vi "HB_ObjectManager.Main.vi"() -> ()   [LabVIEW 2009, in "HB_BaseClass_Examples.lvlib"]
doc: "Demo VI to demonstrate the usage of the HGF_ObjectManager."
uses:
  HB_BaseClass_Examples.lvlib
  HB_Factory/HB_Factory.lvclass
  lib.lib/HGF_LVC/HGF_ObjectManager/HGF_ObjectManager.lvlib
  lib.lib/HGF_LVC/HGF_BaseClasses/HGF_Reference/HGF_Reference.lvclass
  HB_Simple/HB_Simple.lvclass
  lib.lib/HGF_LVC/HGF_Auxiliary/HGF_Auxiliary.lvlib
panel:
  out "values":dbl[](array[numeric])
  in  "stop":bool
  out "initDataFound":bool
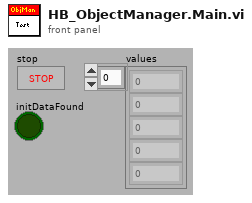
[diagram p1: front panel]
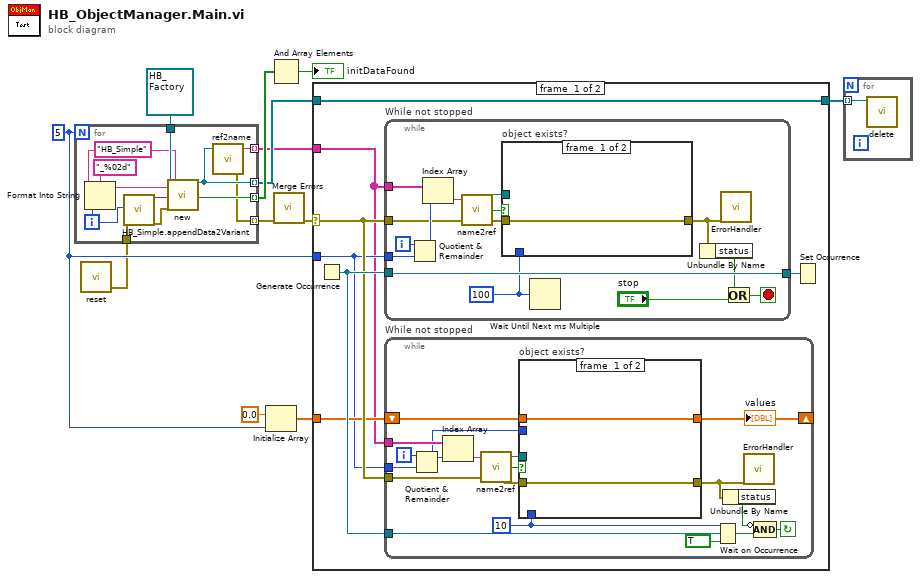
[diagram p0: block diagram]
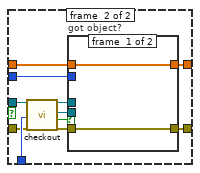
[diagram p2: hidden frame]
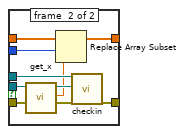
[diagram p3: hidden frame]
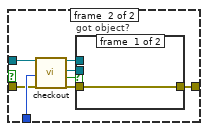
[diagram p4: hidden frame]
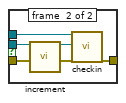
[diagram p5: hidden frame]
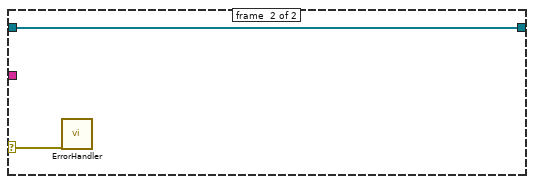
[diagram p6: hidden frame]
diagram:
  w4 = 5
  n1 = call "reset.vi"() -> ("error out"=w1:errorcluster)  [unwired: 1 in, 4 out]
  n2 = for {
    N: w4 -> [_]
    tunnel: refnum<class "HB_Factory.lvclass"> refnum ("HB_HGF_Test.lvlib:HB_Factory.lvclass") -> [w22]
    tunnel: [w17] -> w8 mode=indexing
    tunnel: [w16] -> w9 mode=indexing
    tunnel: [w19] -> w11 mode=indexing
    tunnel: [w15] -> w2 mode=indexing
    tunnel: w1 -> [w13]
    i -> [w23]
    w21 = "HB_Simple" ("className")
    n3 = Format Into String(format string="_%02d", initial string=w21, w23) -> (resulting string=w18:string)  [unwired: 1 in, 1 out]
    n4 = call "HB_Simple.appendData2Variant.vi"("x"=w23, "error in (no error)"=w13) -> ("dup initData"=w20:variant, "error out"=w14:errorcluster)  [unwired: 16 in]
    n5 = call "new.vi"("HGF_Factory"=w22, "objectName"=w18, "initializationData"=w20, "error in (no error)"=w14, "className"=w21) -> ("objectRef"=w17:refnum<class "HGF_Reference.lvclass">, "found?"=w19:bool)  [unwired: 4 in, 9 out]
    n6 = call "ref2name.vi"("objectRef"=w17) -> ("error out"=w16:errorcluster, "name out"=w15:string)  [unwired: 1 in, 2 out]
  }
  n7 = Initialize Array(0.0 ("element"), w4) -> (w3:dbl[])
  n8 = And Array Elements(Boolean array=w11) -> (logical AND=→"initDataFound":bool)
  n9 = call <vilib>:"Merge Errors.vi"("error array in"=w9) -> ("error out"=w6:errorcluster)  [unwired: 3 in, 3 out]
  n10 = case shown="No Error" w6 {
    selector: w6 -> [w29 w106]
    tunnel: w4 -> [w27 _]
    tunnel: w8 -> [w25 w107]
    tunnel: [w25 w107] -> w7
    tunnel: w3 -> [w28 _]
    tunnel: w2 -> [w26 _]
    frame #0 {
      n11 = Generate Occurrence() -> (w30:refnum<k4>)
      n12 = while "While not stopped" {
        tunnel: w27 -> [w88]
        tunnel: w26 -> [w87]
        tunnel: w29 -> [w78]
        tunnel: w30 -> [w85]
        tunnel: [w85] -> w31
        i -> [w89]
        stop <- w82 stop-if-true
        w80 = u32 100 ("millisecond multiple")
        n13 = Quotient & Remainder(x=w89, y=w88) -> (x-y*floor(x/y)=w86:i32)  [unwired: 1 out]
        n14 = Index Array(array=w87, index=w86) -> (element=w79:string)
        n15 = call "name2ref.vi"("error in (no error)"=w78, "name"=w79) -> ("error out"=w77:errorcluster, "obj exists"=w75:bool, "objectRef out"=w76:refnum<class "HGF_Reference.lvclass">)  [unwired: 1 out]
        n16 = case "object exists?" shown="True" w75 {
          tunnel: [w90 w94] -> w81
          tunnel: w80 -> [_ w93]
          tunnel: w77 -> [w90 w92]
          tunnel: w76 -> [_ w91]
          frame #0 {
          }
          frame #1 {
            n17 = call "checkout.vi"("HGF_Reference"=w91, "timeout in ms (-1)"=w93, "error in (no error)"=w92) -> ("dup HGF_Reference"=w96:refnum<class "HGF_Reference.lvclass">, "HB_Simple"=w95:refnum<class "HB_Simple.lvclass">, "got object?"=w98:bool, "error out"=w97:errorcluster)  [unwired: 13 in]
            n18 = case "got object?" shown="True" w98 {
              tunnel: w95 -> [_ w104]
              tunnel: w96 -> [_ w105]
              tunnel: w97 -> [w99 w102]
              tunnel: [w99 w100] -> w94
              frame #0 {
              }
              frame #1 {
                n19 = call "increment.vi"("HB_Simple in"=w104, "error in (no error)"=w102) -> ("HB_Simple out"=w103:refnum<class "HB_Simple.lvclass">, "error out"=w101:errorcluster)  [unwired: 16 out]
                n20 = call "checkin.vi"("HGF_Reference"=w105, "Object"=w103, "error in (no error)"=w101) -> ("error out"=w100:errorcluster)  [unwired: 1 in, 15 out]
              }
            }
          }
        }
        n21 = Wait Until Next ms Multiple(millisecond multiple=w80) -> ()  [unwired: 1 out]
        n22 = Unbundle By Name(w81) -> ("status"=w84:bool)
        n23 = call "ErrorHandler.vi"("error in (no error)"=w81) -> ()  [unwired: 6 in, 13 out]
        n24 = Or(x=w84, y="stop") -> (x .or. y?=w82:bool)
      }
      n25 = while "While not stopped" {
        tunnel: w26 -> [w45]
        tunnel: w29 -> [w34]
        tunnel: w30 -> [w48]
        shift-right: [w39] -> _
        shift-left: w28 -> [w41]
        tunnel: w27 -> [w38]
        i -> [w49]
        stop <- w42 continue-if-true
        w47 = 10 ("timeout in ms (-1)")
        n26 = Quotient & Remainder(x=w49, y=w38) -> (x-y*floor(x/y)=w40:i32)  [unwired: 1 out]
        n27 = Index Array(array=w45, index=w40) -> (element=w35:string)
        n28 = call "name2ref.vi"("error in (no error)"=w34, "name"=w35) -> ("error out"=w33:errorcluster, "obj exists"=w32:bool, "objectRef out"=w36:refnum<class "HGF_Reference.lvclass">)  [unwired: 1 out]
        n29 = case "object exists?" shown="True" w32 {
          tunnel: w47 -> [_ w58]
          tunnel: w41 -> [w51 w57]
          tunnel: w40 -> [_ w56]
          tunnel: [w51 w55] -> w39
          tunnel: [w50 w54] -> w37
          tunnel: w36 -> [_ w53]
          tunnel: w33 -> [w50 w52]
          frame #0 {
          }
          frame #1 {
            n30 = call "checkout.vi"("HGF_Reference"=w53, "timeout in ms (-1)"=w58, "error in (no error)"=w52) -> ("dup HGF_Reference"=w60:refnum<class "HGF_Reference.lvclass">, "HB_Simple"=w59:refnum<class "HB_Simple.lvclass">, "got object?"=w62:bool, "error out"=w61:errorcluster)  [unwired: 13 in]
            n31 = case "got object?" shown="True" w62 {
              tunnel: w59 -> [_ w72]
              tunnel: w60 -> [_ w74]
              tunnel: w61 -> [w64 w71]
              tunnel: [w64 w73] -> w54
              tunnel: w57 -> [w63 w67]
              tunnel: w56 -> [_ w66]
              tunnel: [w63 w65] -> w55
              frame #0 {
              }
              frame #1 {
                n32 = call "get_x.vi"("HB_Simple"=w72, "error in (no error)"=w71) -> ("dup HB_Simple"=w69:refnum<class "HB_Simple.lvclass">, "x"=w68:dbl, "error out"=w70:errorcluster)  [unwired: 15 out]
                n33 = Replace Array Subset(array=w67, new element=w68, index=w66) -> (w65:dbl[])
                n34 = call "checkin.vi"("HGF_Reference"=w74, "Object"=w69, "error in (no error)"=w70) -> ("error out"=w73:errorcluster)  [unwired: 1 in, 15 out]
              }
            }
          }
        }
        "values" <- w39
        n35 = Wait on Occurrence(1:TRUE ("ignore previous (T)"), 2:w48, 3:w47) -> (0:w43:bool)
        n36 = Unbundle By Name(w37) -> ("status"=w44:bool)
        n37 = call "ErrorHandler.vi"("error in (no error)"=w37) -> ()  [unwired: 6 in, 13 out]
        n38 = Compound Arithmetic op=AND(invert w44, w43) -> (w42:bool)
      }
      n39 = Set Occurrence(w31) -> ()
    }
    frame #1 {
      n40 = call "ErrorHandler.vi"("error in (no error)"=w106) -> ()  [unwired: 6 in, 13 out]
    }
  }
  n41 = for {
    tunnel: w7 -> [w108] mode=indexing
    n42 = call "delete.vi"("objectRef"=w108) -> ()  [unwired: 3 in, 4 out]
  }
